vi "Translate Active Pixels.vi"(8 "error in (no error)":errorcluster, 10 "Enum":enum16{"Move Left", "Don't Move", "Move Right"}(ring), 11 "Game Engine in":refnum<class "Game Engine.lvclass">) -> (0 "error out":errorcluster, 3 "Game Engine out":refnum<class "Game Engine.lvclass">)   [LabVIEW 2017, in "Game Engine.lvlib" / "Game Engine.lvclass"]
uses:
  Game Engine.lvclass
  Game Engine.lvclass/Game Engine.ctl
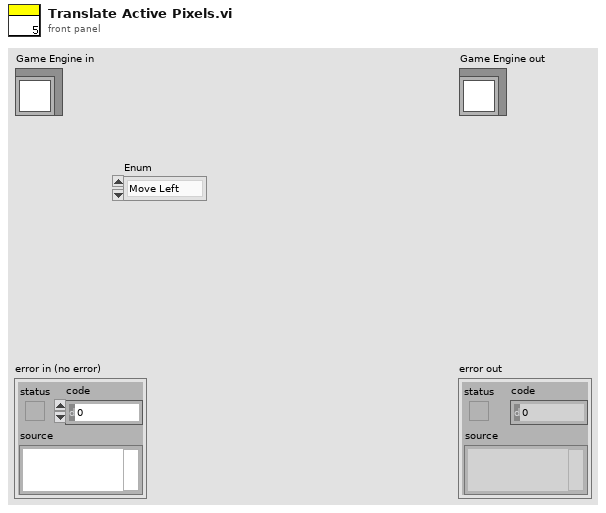
[diagram p1: front panel]
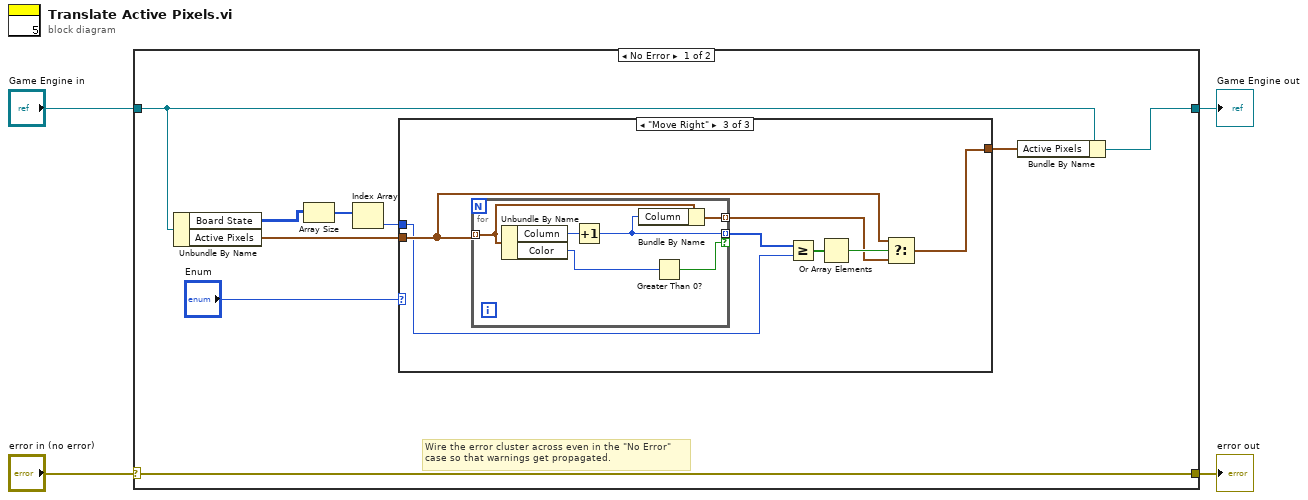
[diagram p0: block diagram]
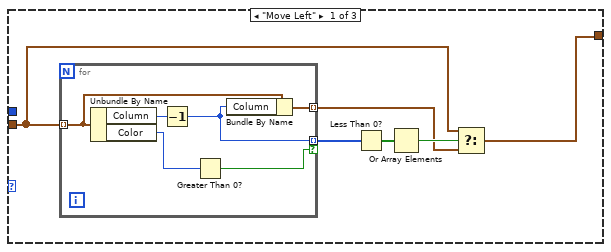
[diagram p2: hidden frame]
diagram:
  n1 = case shown="No Error" "error in (no error)" {
    selector: "error in (no error)" -> [w13 w41]
    tunnel: [w13 w41] -> w3
    tunnel: [w9 w40] -> w1
    tunnel: "Game Engine in" -> [w10 w40]
    frame No Error {
      # "Wire the error cluster across even in the \"No Error\"\ncase so that warnings get propagated."
      n2 = Unbundle By Name(w10) -> ("Board State"=w7:u32[][], "Active Pixels"=w11:cluster{"Column":u8, "Row":u8, "Color":u32}[])
      n3 = Array Size(array=w7) -> (size(s)=w6:i32[])
      n4 = Index Array(array=w6) -> (element=w5:i32)  [unwired: 1 in]
      n5 = case shown="\"Move Right\"" "Enum" {
        tunnel: w11 -> [w16 w26 w31]
        tunnel: [w15 w26 w27] -> w8
        tunnel: w5 -> [_ _ w28]
        frame "Move Left" {
          n6 = for {
            tunnel: w16 -> [w24] mode=indexing
            tunnel: [w23] -> w19 mode=indexing if=w20
            tunnel: [w22] -> w14 mode=indexing
            n7 = Unbundle By Name(w24) -> ("Column"=w25:u8, "Color"=w21:u32)
            n8 = Decrement(x=w25) -> (x-1=w23:u8)
            n9 = Greater Than 0?(x=w21) -> (x > 0?=w20:bool)
            n10 = Bundle By Name(cluster=w24, "Column"=w23) -> (w22:cluster{"Column":u8, "Row":u8, "Color":u32})
          }
          n11 = Less Than 0?(x=w19) -> (x < 0?=w18:bool[])
          n12 = Or Array Elements(Boolean array=w18) -> (logical OR=w17:bool)
          n13 = Select(t=w16, s=w17, f=w14) -> (s? t:f=w15:cluster{"Column":u8, "Row":u8, "Color":u32}[])
        }
        frame "Don't Move", Default {
        }
        frame "Move Right" {
          n14 = for {
            tunnel: w31 -> [w38] mode=indexing
            tunnel: [w37] -> w29 mode=indexing if=w34
            tunnel: [w36] -> w32 mode=indexing
            n15 = Unbundle By Name(w38) -> ("Column"=w39:u8, "Color"=w35:u32)
            n16 = Increment(x=w39) -> (x+1=w37:u8)
            n17 = Bundle By Name(cluster=w38, "Column"=w37) -> (w36:cluster{"Column":u8, "Row":u8, "Color":u32})
            n18 = Greater Than 0?(x=w35) -> (x > 0?=w34:bool)
          }
          n19 = Greater Or Equal?(x=w29, y=w28) -> (x >= y?=w30:bool[])
          n20 = Or Array Elements(Boolean array=w30) -> (logical OR=w33:bool)
          n21 = Select(t=w31, s=w33, f=w32) -> (s? t:f=w27:cluster{"Column":u8, "Row":u8, "Color":u32}[])
        }
      }
      n22 = Bundle By Name(cluster=w10, "Active Pixels"=w8) -> (w9:refnum<class "Game Engine.lvclass">)
    }
    frame Error {
    }
  }
  "error out" <- w3
  "Game Engine out" <- w1
